vi "RT Main.vi"() -> ()   [LabVIEW 2017]
uses:
  Support/Message Queue/Message Cluster.ctl
  Controls/FPGA State.ctl
  Globals/Host/Global - Configuration Options.vi
  Globals/RT/Globals - RT Stream.vi
  Support/Message Queue/Message Queue.lvlib
panel:
  out "Message":string
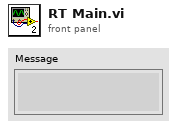
[diagram p1: front panel]
types:
  T1 = typedef "Message Queue.lvlib/All Real-Time Message Queues.ctl" = cluster{"Message Handler":refnum<queue>, "Acquisition and Logging":refnum<queue>}
  T2 = typedef "Message Queue.lvlib/Message Cluster.ctl" = cluster{"Message":string, "Message Data":variant}
  T3 = typedef "FPGA State.ctl" = enum16{"Manual", "Standby", "Automated Sequence", "Automated Sequence End", "Emergency"}
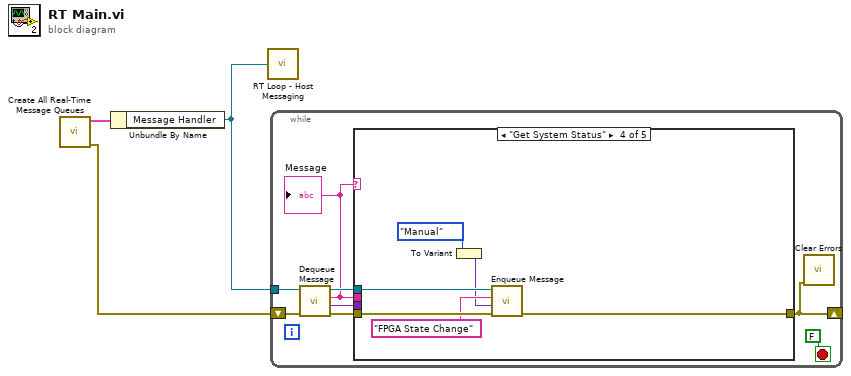
[diagram p0: block diagram]
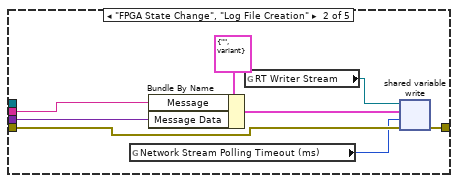
[diagram p3: hidden frame]
diagram:
  n1 = call "Create All Real-Time Message Queues.vi"() -> ("error out"=w1:errorcluster, "Message Queues out"=w3:T1)  [unwired: 10 in]
  n2 = Unbundle By Name(w3) -> ("Message Handler"=w2:refnum<queue>)
  n3 = call "RT Loop - Host Messaging.vi"("Message Queue"=w2) -> ()
  n4 = while {
    tunnel: w2 -> [w11]
    shift-right: [w4] -> _
    shift-left: w1 -> [w5]
    stop <- FALSE stop-if-true
    n5 = call "Dequeue Message.vi"("error in (no error)"=w5, "Message Queue"=w11) -> ("error out"=w10:errorcluster, "Message Data"=w8:variant, "Message"=w7:string, "dup Message Queue"=w9:refnum<queue>)  [unwired: 6 in]
    "Message" <- w7
    n6 = case shown="\"Get System Status\"" w7 {
      tunnel: w10 -> [w12 w17 w21 w26 w28]
      tunnel: w9 -> [_ _ _ w27 _]
      tunnel: w7 -> [_ w20 _ _ _]
      tunnel: w8 -> [_ w13 _ _ _]
      tunnel: [w12 w14 w21 w24 w28] -> w4
      frame "Initialize" {
      }
      frame "FPGA State Change", "Log File Creation" {
        n7 = global read "Global - Configuration Options.vi" "Network Stream Polling Timeout (ms)"() -> (w16:i32)
        n8 = Bundle By Name(cluster=T2 {"Message"="", "Message Data"=variant} ("Message Cluster"), "Message"=w20, "Message Data"=w13) -> (w19:T2)
        n9 = global read "Globals - RT Stream.vi" "RT Writer Stream"() -> (w15:refnum<k21>)
        n10 = shared-variable-write(w15, w17, w19, w16) -> (w14:errorcluster)  [unwired: 2 out]
      }
      frame "--------------" {
      }
      frame "Get System Status" {
        n11 = To Variant(anything=FPGA_State."Manual" ("FPGA States")) -> (Variant=w22:variant)
        n12 = call "Enqueue Message.vi"("error in (no error)"=w26, "Message Data"=w22, "Message"="FPGA State Change", "Message Queue"=w27) -> ("error out"=w24:errorcluster)  [unwired: 6 in, 1 out]
      }
      frame Default {
      }
    }
    n13 = call <vilib>:"Clear Errors.vi"("error in (no error)"=w4) -> ()  [unwired: 5 in, 2 out]
  }
